vi "send_to_process.vi"(8 "error in":errorcluster, 9 "Control_process_state_cluster in":T1={"Control_process_state_enum"=enum."Custom", "variant"=variant}, 10 "Process name":string, 11 "Process_communication in":variant) -> (0 "error out":errorcluster, 3 "Process_communication out":variant)   [LabVIEW 2011, in "Fiberscope_library.lvlib"]
uses:
  Fiberscope_library.lvlib
  typedefs/control_process_state_cluster.ctl
  typedefs/control_process_state_enum.ctl
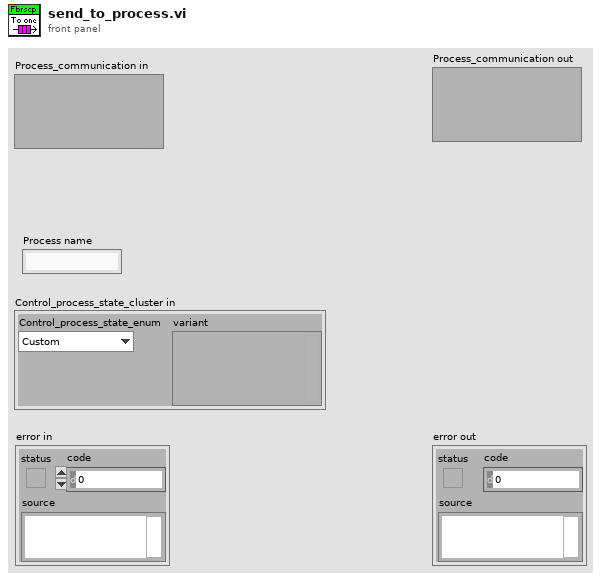
[diagram p1: front panel]
types:
  T1 = typedef "Fiberscope_library.lvlib/control_process_state_cluster.ctl" = cluster{"Control_process_state_enum":T2, "variant":variant}
  T2 = typedef "Fiberscope_library.lvlib/control_process_state_enum.ctl" = enum16{"Init", "Quit", "Start", "Stop", "Change_parameters", "Running", "Finish", "Custom"}
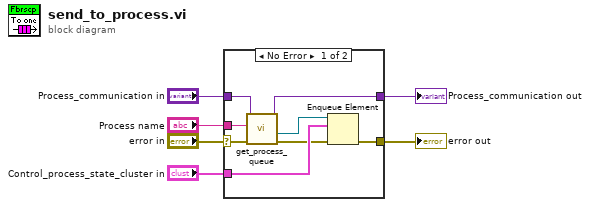
[diagram p0: block diagram]
diagram:
  n1 = case shown="No Error" "error in" {
    selector: "error in" -> [w13 w16]
    tunnel: [w7 w16] -> w5
    tunnel: "Control_process_state_cluster in" -> [w14 _]
    tunnel: "Process_communication in" -> [w12 w15]
    tunnel: "Process name" -> [w9 _]
    tunnel: [w8 w15] -> w1
    frame No Error {
      n2 = call "get_process_queue.vi"("error in (no error)"=w13, "Process name"=w9, "Process_communication in"=w12) -> ("error out"=w11:errorcluster, "Process_control_queue"=w10:refnum<queue>, "Process_communication out"=w8:variant)  [unwired: 6 in]
      n3 = Enqueue Element(queue=w10, element=w14, error in (no error)=w11) -> (error out=w7:errorcluster)  [unwired: 1 in, 2 out]
    }
    frame Error {
    }
  }
  "error out" <- w5
  "Process_communication out" <- w1
